vi "autonSample.vi"(0 "Auton Array":dbl[][](array[numeric]), 5 "MeasuredHeading":dbl, 9 "EncoderDistance":dbl) -> (4 "Left Drive":dbl(knob) scale=-1.0..1.0, 6 "Right Drive":dbl(knob) scale=-1.0..1.0, 8 "Ramp ACT motor":dbl, 10 "Turret Rotation":dbl, 13 "Conveyor":dbl, 14 "Harvester":dbl, 15 "Shooter motor output":dbl)   [LabVIEW 2011]
uses:
  Robot Global Data.vi
  <vilib>/addons/control/pid/pid.llb/PID (DBL).vi
  <vilib>/addons/control/pid/NI_PID_pid.lvlib
panel:
  out "Numeric":i16
  out "Tzero":i64
  out "AccumDist":dbl
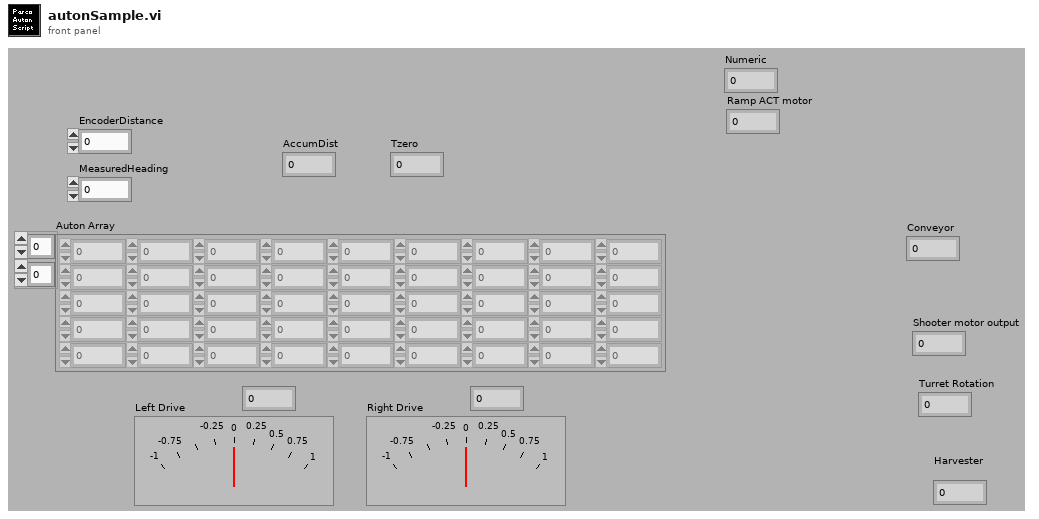
[diagram p1: front panel]
types:
  T1 = cluster{"proportional gain (Kc)":dbl, "integral time (Ti, min)":dbl, "derivative time (Td, min)":dbl}
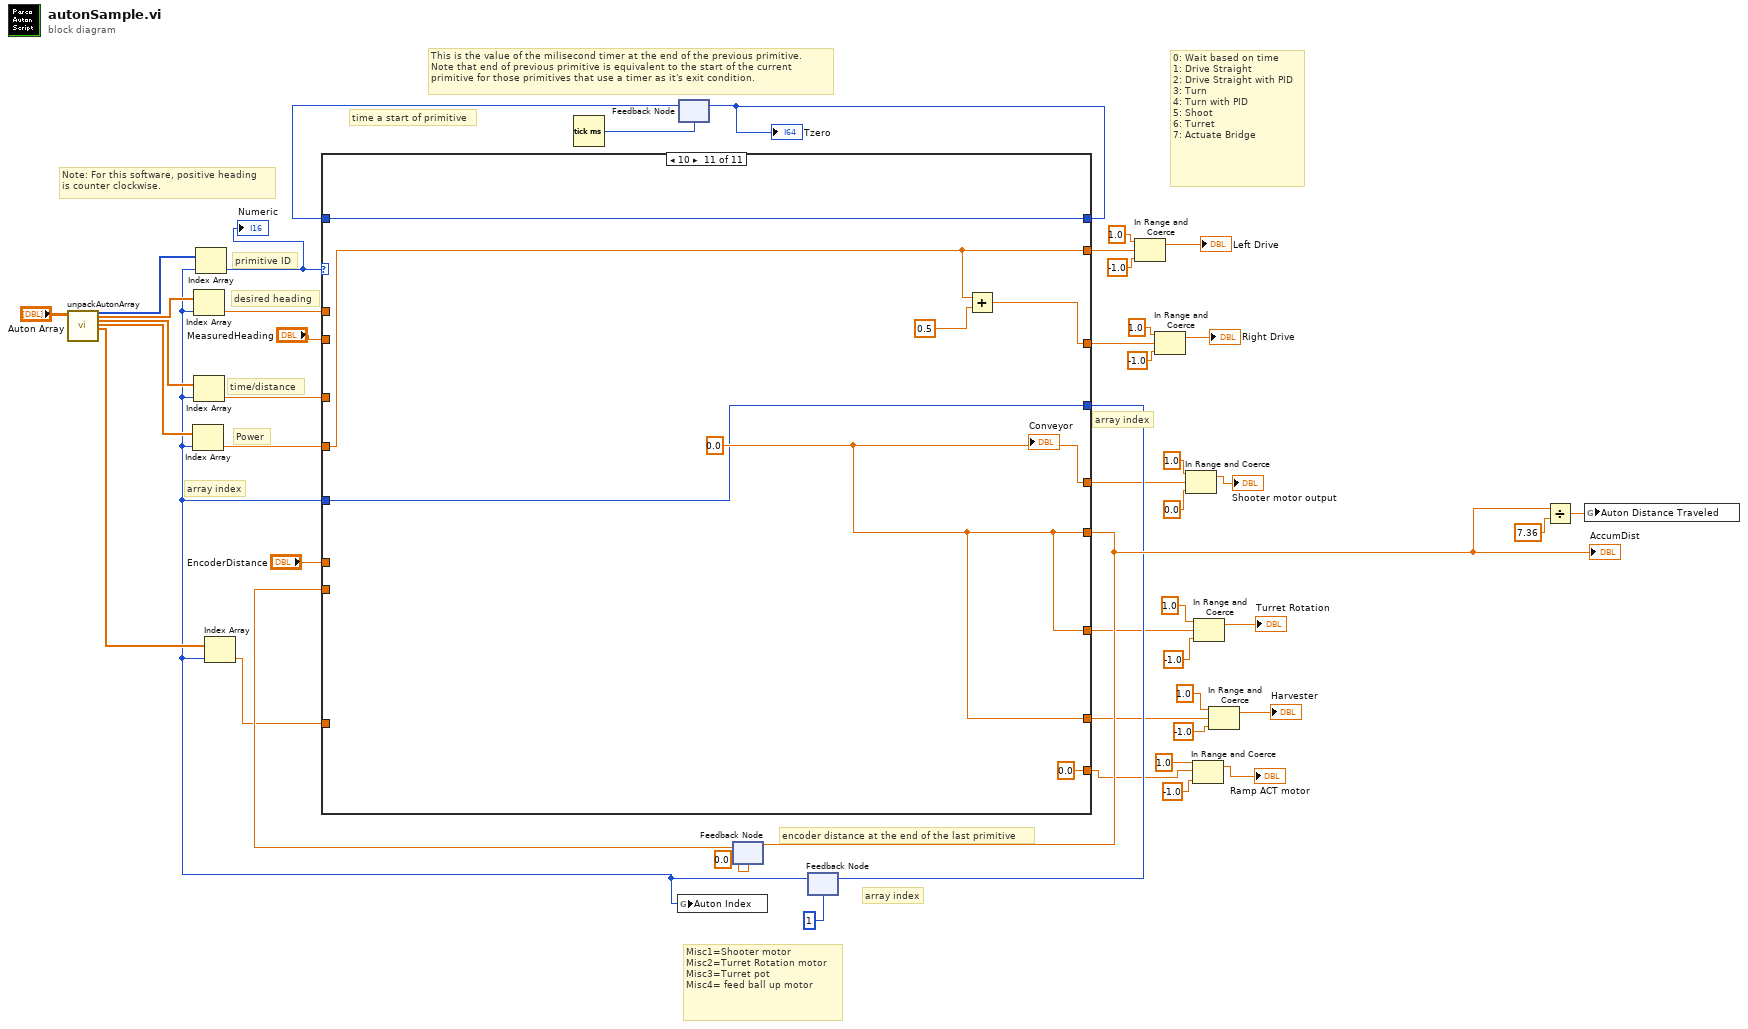
[diagram p0: block diagram]
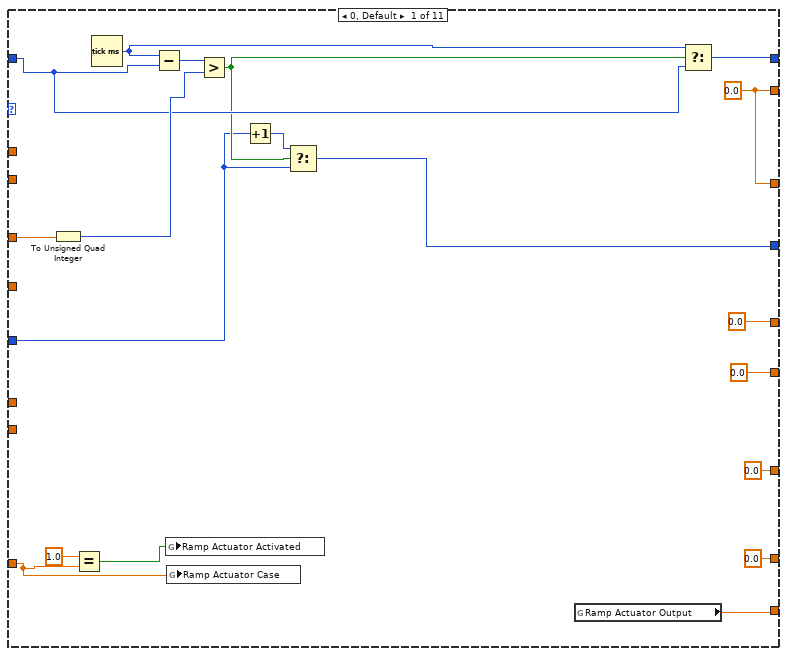
[diagram p2: hidden frame]
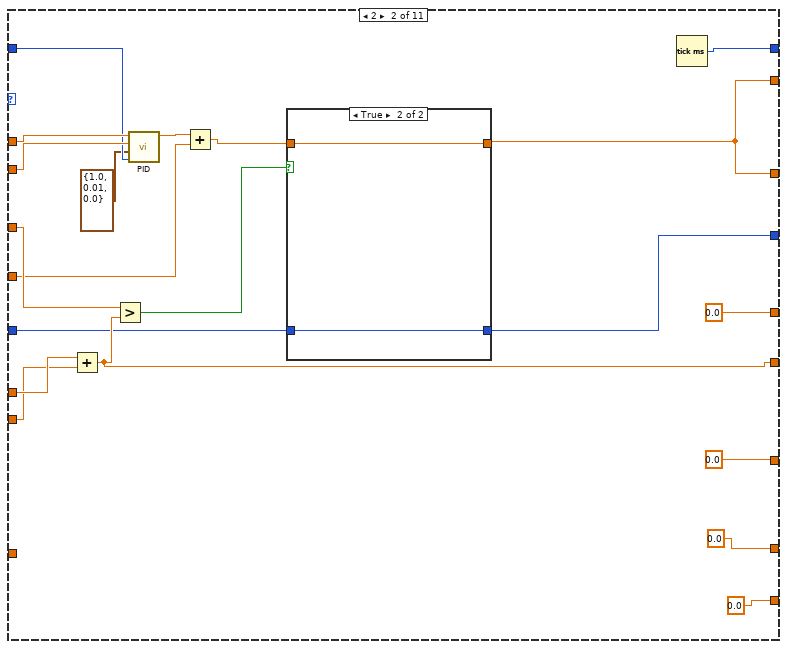
[diagram p3: hidden frame]
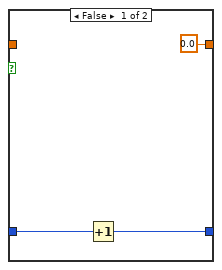
[diagram p4: hidden frame]
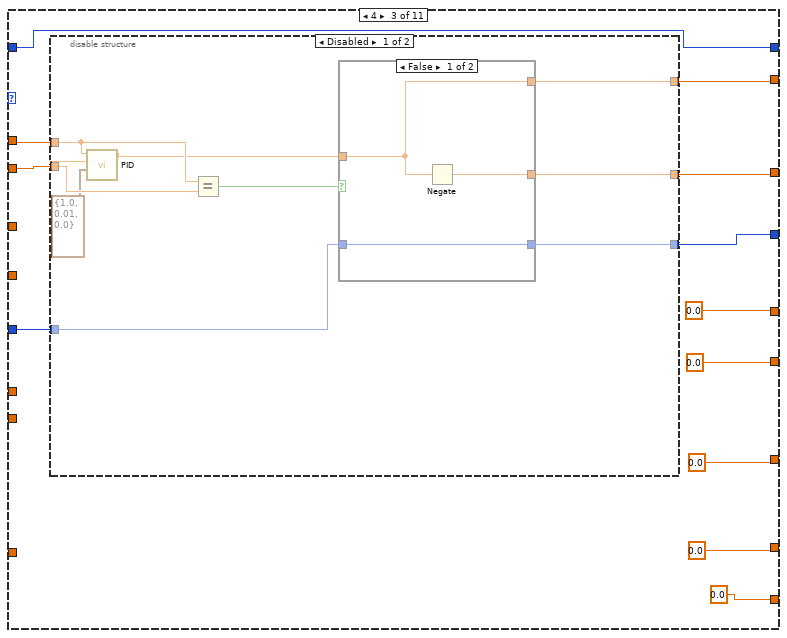
[diagram p5: hidden frame]
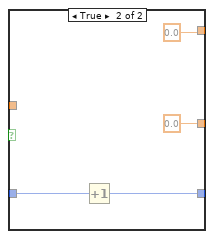
[diagram p6: hidden frame]
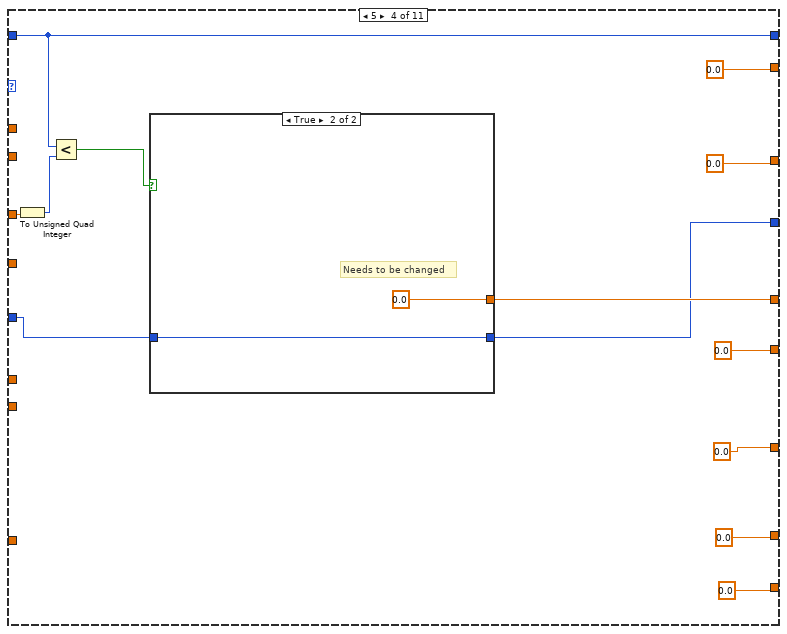
[diagram p8: hidden frame]
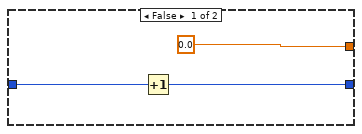
[diagram p9: hidden frame]
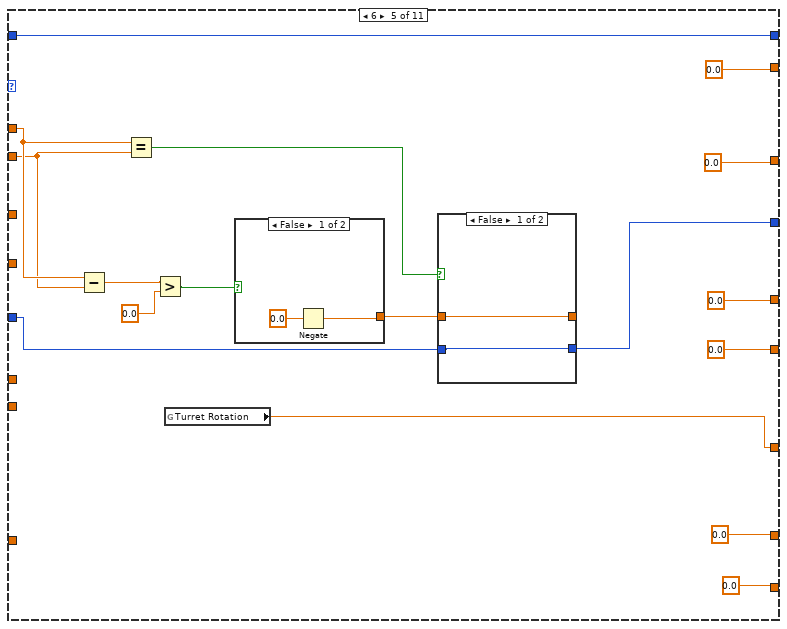
[diagram p10: hidden frame]
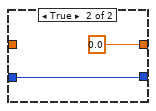
[diagram p11: hidden frame]
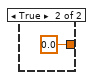
[diagram p12: hidden frame]
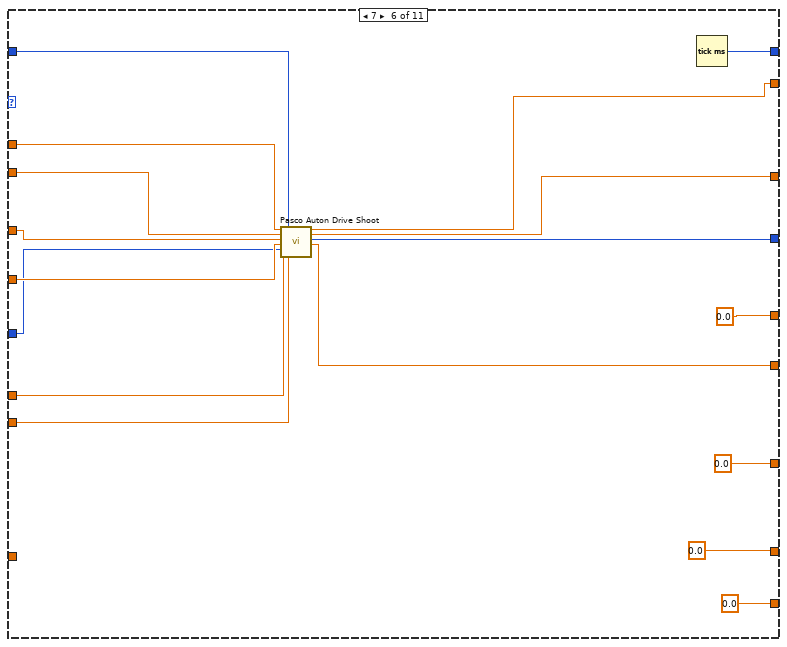
[diagram p13: hidden frame]
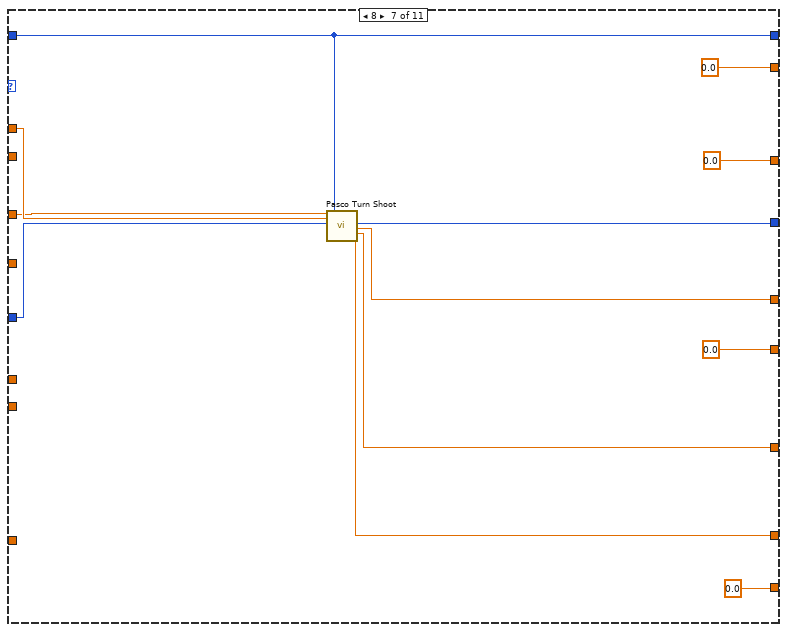
[diagram p14: hidden frame]
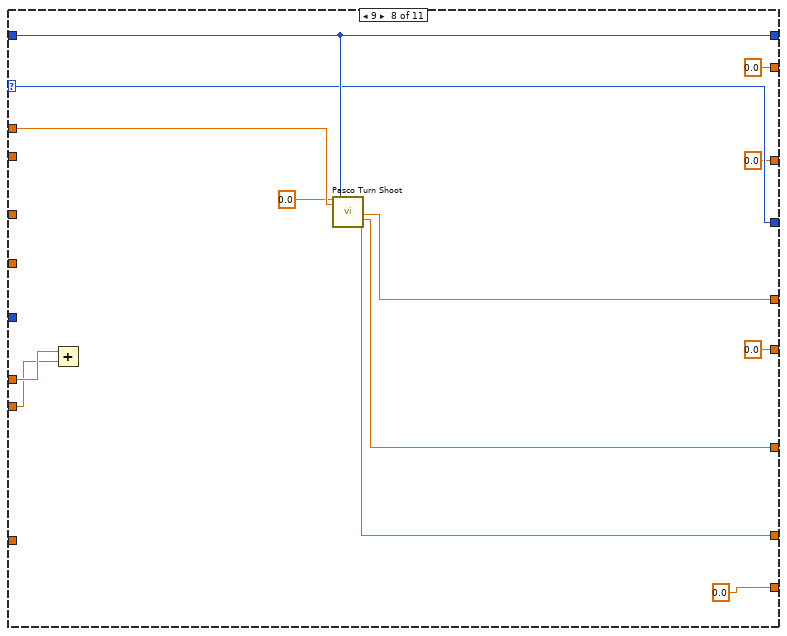
[diagram p15: hidden frame]
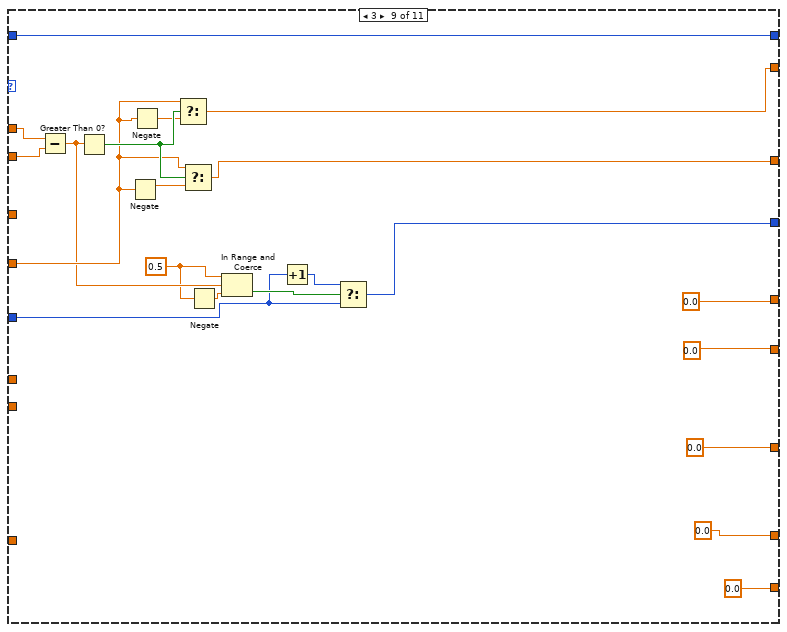
[diagram p16: hidden frame]
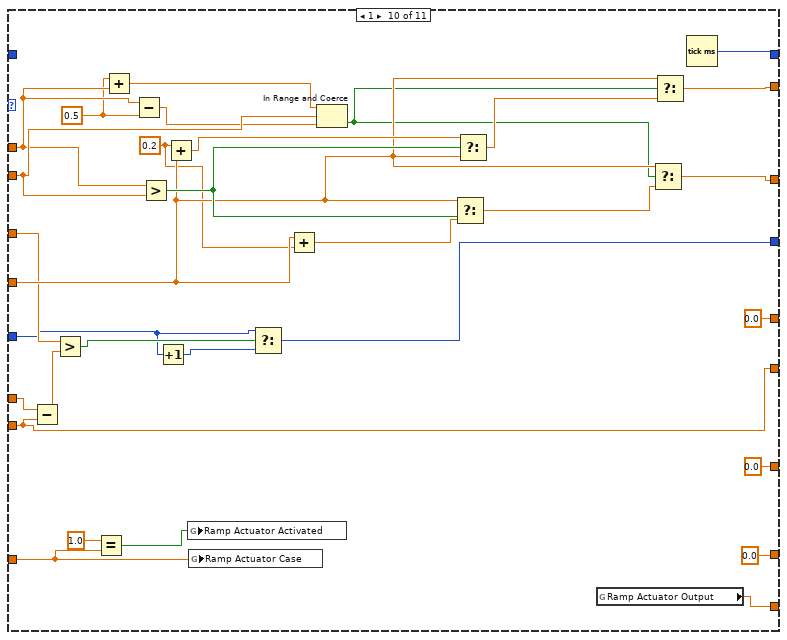
[diagram p17: hidden frame]
diagram:
  # "Misc1=Shooter motor\nMisc2=Turret Rotation motor\nMisc3=Turret pot\nMisc4= feed ball up motor"
  # "0: Wait based on time\n1: Drive Straight\n2: Drive Straight with PID\n3: Turn\n4: Turn with PID\n5: Shoot\n6: Turret\n7: Actuate Bridge"
  # "encoder distance at the end of the last primitive"
  # "Note: For this software, positive heading\nis counter clockwise."
  # "time a start of primitive"
  # "array index"
  # "array index"
  # "This is the value of the milisecond timer at the end of the previous primitive.\nNote that end of previous primitive is equivalent to the start of the current\nprimitive for those primitives that use a timer as it's exit condition."
  # "Power"
  # "array index"
  # "desired heading"
  # "primitive ID"
  # "time/distance"
  n1 = call "unpackAutonArray.vi"("all rows"="Auton Array") -> ("Primitive"=w47:i16[], "Left Drive"=w30:dbl[], "Right Drive"=w31:dbl[], "Ramp ACT"=w28:dbl[], "Conveyor"=w7:dbl[])  [unwired: 1 in, 21 out]
  n2 = Tick Count (ms)() -> (millisecond timer value=w42:u32)
  n3 = feedback #1(w42) -> (w46:u32)
  n4 = feedback #2(0.0 ("EncoderDistance")) -> (w27:dbl)
  n5 = feedback #3(1) -> (w6:i32)
  n6 = Index Array(array=w28, index=w6) -> (element=w44:dbl)
  n7 = Index Array(array=w30, index=w6) -> (element=w29:dbl)
  n8 = Index Array(array=w31, index=w6) -> (element=w45:dbl)
  n9 = Index Array(array=w47, index=w6) -> (element=w8:i16)
  "Numeric" <- w8
  n10 = Index Array(array=w7, index=w6) -> (element=w5:dbl)
  n11 = case shown="10" w8 {
    selector: w8 -> [_ _ _ _ _ _ _ w195 _ _ _]
    tunnel: [w55 w80 w98 w128 w151 w164 w188 w195 w207 w236 w262] -> w22
    tunnel: w6 -> [w56 w81 w97 w129 w152 w171 w191 _ w209 w234 w262]
    tunnel: [w67 w87 w104 w123 w150 w177 w189 w199 w205 w255 w261] -> w32
    tunnel: w46 -> [w63 w74 w104 w123 w150 w168 w189 w199 w205 _ w261]
    tunnel: w45 -> [w65 w83 _ w133 _ w173 w185 _ _ w238 _]
    tunnel: w29 -> [_ w75 w94 _ w155 w175 w190 w202 w221 w248 _]
    tunnel: [w54 w82 w99 0.0 0.0 w167 0.0 0.0 ("Numeric") w215 w239 w259] -> w40
    tunnel: [w54 w82 w100 0.0 0.0 w166 0.0 0.0 ("Right Drive") w214 w240 w258] -> w33
    tunnel: w44 -> [_ w71 _ _ _ w172 _ _ w217 w243 w259]
    tunnel: "EncoderDistance" -> [_ w86 _ _ _ w169 _ w204 _ w233 _]
    tunnel: "MeasuredHeading" -> [_ w76 w95 _ w141 w174 _ _ w220 w249 _]
    tunnel: [0.0 ("Encoder total") w84 0.0 0.0 0.0 w165 0.0 0.0 ("Encoder total") 0.0 w231 w263] -> w24
    tunnel: w27 -> [_ w85 _ _ _ w170 _ w203 _ w231 _]
    tunnel: [0.0 ("Misc1  OUT") 0.0 0.0 w130 0.0 0.0 ("Misc1  OUT") w187 w201 0.0 0.0 ("Misc1  OUT") w263] -> w18
    tunnel: [0.0 ("Misc2 OUT") 0.0 0.0 0.0 w140 0.0 ("Misc1  OUT") w186 w200 0.0 0.0 ("Misc2 OUT") w263] -> w14
    tunnel: [0.0 ("Misc4 OUT") 0.0 0.0 0.0 0.0 0.0 w181 w197 0.0 0.0 w263] -> w10
    tunnel: w5 -> [w50 _ _ _ _ _ _ _ _ w229 _]
    tunnel: [w49 0.0 ("Ramp Actuator Output") 0.0 ("Ramp Actuator Output") 0.0 ("Ramp Actuator Output") 0.0 ("Ramp Actuator Output") 0.0 ("Ramp Actuator Output") 0.0 ("Ramp Actuator Output") 0.0 ("Ramp Actuator Output") 0.0 ("Ramp Actuator Output") w226 0.0 ("Ramp Actuator Output")] -> w4
    frame 0, Default {
      w54 = 0.0 ("Numeric")
      n12 = To Unsigned Quad Integer(1:w65) -> (0:w64:u64)
      n13 = Equal?(x=1.0, y=w50) -> (x = y?=w51:bool)
      n14 = Tick Count (ms)() -> (millisecond timer value=w62:u32)
      n15 = Subtract(x=w62, y=w63) -> (x-y=w66:u32)
      n16 = global write "Robot Global Data.vi" "Ramp Actuator Activated"(w51) -> ()
      n17 = global write "Robot Global Data.vi" "Ramp Actuator Case"(w50) -> ()
      n18 = Greater?(x=w66, y=w64) -> (0:w58:bool)
      n19 = Increment(x=w56) -> (x+1=w57:i32)
      n20 = Select(t=w57, s=w58, f=w56) -> (s? t:f=w55:i32)
      n21 = global read "Robot Global Data.vi" "Ramp Actuator Output"() -> (w49:dbl)
      n22 = Select(t=w62, s=w58, f=w63) -> (s? t:f=w67:u32)
    }
    frame 2 {
      n23 = Add(x=w86, y=w85) -> (x+y=w84:dbl)
      n24 = Greater?(x=w83, y=w84) -> (0:w73:bool)
      n25 = call-poly <vilib>:"PID.vi"("dt (s)"=w74, "PID gains"=T1 {"proportional gain (Kc)"=1.0, "integral time (Ti, min)"=0.01, "derivative time (Td, min)"=0.0}, "process variable"=w76, "setpoint"=w75) -> ("output"=w70:dbl)  [unwired: 6 in, 1 out]
      n26 = Add(x=w70, y=w71) -> (x+y=w69:dbl)
      n27 = case shown="True" w73 {
        tunnel: [0.0 w92] -> w82
        tunnel: w69 -> [_ w92]
        tunnel: w81 -> [w90 w91]
        tunnel: [w89 w91] -> w80
        frame False {
          n28 = Increment(x=w90) -> (x+1=w89:i32)
        }
        frame True {
        }
      }
      n29 = Tick Count (ms)() -> (millisecond timer value=w87:u32)
    }
    frame 4 {
      n30 = disable-structure shown="Disabled" {
        disable-tunnel: [w113 _] -> w100
        disable-tunnel: [w112 _] -> w99
        disable-tunnel: [w111 _] -> w98
        disable-tunnel: w97 -> [w110 _]
        disable-tunnel: w95 -> [w108 _]
        disable-tunnel: w94 -> [w107 _]
        frame Disabled {
          n31 = call-poly <vilib>:"PID.vi"("PID gains"=T1 {"proportional gain (Kc)"=1.0, "integral time (Ti, min)"=0.01, "derivative time (Td, min)"=0.0}, "process variable"=w108, "setpoint"=w107) -> ("output"=w106:dbl)  [unwired: 7 in, 1 out]
          n32 = Equal?(x=w107, y=w108) -> (x = y?=w109:bool)
          n33 = case shown="False" w109 {
            tunnel: w106 -> [w115 _]
            tunnel: [w116 0.0] -> w113
            tunnel: [w115 0.0] -> w112
            tunnel: [w114 w119] -> w111
            tunnel: w110 -> [w114 w120]
            frame False {
              n34 = Negate(x=w115) -> (-x=w116:dbl)
            }
            frame True {
              n35 = Increment(x=w120) -> (x+1=w119:i32)
            }
          }
        }
        frame Enabled {
        }
      }
    }
    frame 5 {
      n36 = To Unsigned Quad Integer(1:w133) -> (0:w131:u64)
      n37 = Less?(x=w123, y=w131) -> (x < y?=w132:bool)
      n38 = case shown="True" w132 {
        tunnel: [0.0 0.0] -> w130
        tunnel: w129 -> [w135 w138]
        tunnel: [w134 w138] -> w128
        frame False {
          n39 = Increment(x=w135) -> (x+1=w134:i32)
        }
        frame True {
          # "Needs to be changed"
        }
      }
    }
    frame 6 {
      n40 = Subtract(x=w155, y=w141) -> (x-y=w143:dbl)
      n41 = Equal?(x=w155, y=w141) -> (x = y?=w154:bool)
      n42 = Greater?(x=w143, y=0.0) -> (0:w144:bool)
      n43 = global read "Robot Global Data.vi" "Turret Rotation"() -> (w140:dbl)
      n44 = case shown="False" w144 {
        tunnel: [w161 0.0] -> w153
        frame False {
          n45 = Negate(x=0.0) -> (-x=w161:dbl)
        }
        frame True {
        }
      }
      n46 = case shown="False" w154 {
        tunnel: [w157 0.0] -> _
        tunnel: w153 -> [w157 _]
        tunnel: w152 -> [w156 w159]
        tunnel: [w156 w159] -> w151
        frame False {
        }
        frame True {
        }
      }
    }
    frame 7 {
      n47 = call "Pasco Auton Drive Shoot.vi"("Desired Heading"=w175, "Actual Heading"=w174, "time/distance"=w173, "Power"=w172, "Array"=w171, "Encoder total"=w169, "Time"=w168, "Encoder Return"=w170) -> ("Left Drive"=w167:dbl, "Right Drive"=w166:dbl, "Array Out"=w164:i32, "Encoder total"=w165:dbl)  [unwired: 8 in]
      n48 = Tick Count (ms)() -> (millisecond timer value=w177:u32)
    }
    frame 8 {
      n49 = call "Pasco Turn Shoot.vi"("time/distance"=w185, "desired heading"=w190, "array index"=w191, "primitive time"=w189) -> ("array index"=w188:i32, "Misc1  OUT"=w187:dbl, "Misc2 OUT"=w186:dbl, "Misc4 OUT"=w181:dbl)  [unwired: 12 in]
    }
    frame 9 {
      n50 = Add(x=w204, y=w203) -> ()  [unwired: 1 out]
      n51 = call "Pasco Turn Shoot.vi"("time/distance"=0.0, "desired heading"=w202, "primitive time"=w199) -> ("Misc1  OUT"=w201:dbl, "Misc2 OUT"=w200:dbl, "Misc4 OUT"=w197:dbl)  [unwired: 13 in, 1 out]
    }
    frame 3 {
      w212 = 0.5 ("upper limit")
      n52 = Subtract(x=w221, y=w220) -> (x-y=w213:dbl)
      n53 = Greater Than 0?(x=w213) -> (x > 0?=w219:bool)
      n54 = Negate(x=w217) -> (-x=w218:dbl)
      n55 = Negate(x=w217) -> (-x=w216:dbl)
      n56 = Select(t=w217, s=w219, f=w216) -> (s? t:f=w215:dbl)
      n57 = Select(t=w217, s=w219, f=w218) -> (s? t:f=w214:dbl)
      n58 = Negate(x=w212) -> (-x=w211:dbl)
      n59 = In Range and Coerce(upper limit=w212, x=w213, lower limit=w211) -> (In Range?=w210:bool)  [unwired: 1 out]
      n60 = Increment(x=w209) -> (x+1=w208:i32)
      n61 = Select(t=w208, s=w210, f=w209) -> (s? t:f=w207:i32)
    }
    frame 1 {
      w247 = 0.5 ("x")
      w230 = 0.2 ("x")
      n62 = Subtract(x=w233, y=w231) -> (x-y=w232:dbl)
      n63 = Greater?(x=w238, y=w232) -> (0:w237:bool)
      n64 = Equal?(x=1.0, y=w229) -> (x = y?=w227:bool)
      n65 = Add(x=w247, y=w248) -> (x+y=w245:dbl)
      n66 = Subtract(x=w248, y=w247) -> (x-y=w246:dbl)
      n67 = Greater?(x=w248, y=w249) -> (0:w251:bool)
      n68 = Increment(x=w234) -> (x+1=w235:i32)
      n69 = Add(x=w230, y=w243) -> (x+y=w252:dbl)
      n70 = global write "Robot Global Data.vi" "Ramp Actuator Activated"(w227) -> ()
      n71 = global write "Robot Global Data.vi" "Ramp Actuator Case"(w229) -> ()
      n72 = Select(t=w234, s=w237, f=w235) -> (s? t:f=w236:i32)
      n73 = Add(x=w243, y=w230) -> (x+y=w250:dbl)
      n74 = In Range and Coerce(upper limit=w245, x=w249, lower limit=w246) -> (In Range?=w242:bool)  [unwired: 1 out]
      n75 = Select(t=w243, s=w251, f=w250) -> (s? t:f=w241:dbl)
      n76 = Select(t=w252, s=w251, f=w243) -> (s? t:f=w244:dbl)
      n77 = global read "Robot Global Data.vi" "Ramp Actuator Output"() -> (w226:dbl)
      n78 = Select(t=w243, s=w242, f=w241) -> (s? t:f=w240:dbl)
      n79 = Select(t=w243, s=w242, f=w244) -> (s? t:f=w239:dbl)
      n80 = Tick Count (ms)() -> (millisecond timer value=w255:u32)
    }
    frame 10 {
      w263 = 0.0
      n81 = Add(x=w259, y=0.5 ("x+y")) -> (x+y=w258:dbl)
    }
  }
  "AccumDist" <- w24
  "Tzero" <- w32
  n82 = global write "Robot Global Data.vi" "Auton Index"(w6) -> ()
  n83 = feedback-in #1(w32) -> ()
  n84 = feedback-in #2(w24) -> ()
  n85 = feedback-in #3(w22) -> ()
  n86 = In Range and Coerce(upper limit=1.0, x=w40, lower limit=-1.0) -> (coerced(x)=→"Left Drive":dbl)  [unwired: 1 out]
  n87 = In Range and Coerce(upper limit=1.0, x=w33, lower limit=-1.0) -> (coerced(x)=→"Right Drive":dbl)  [unwired: 1 out]
  n88 = In Range and Coerce(upper limit=1.0, x=w18, lower limit=0.0) -> (coerced(x)=→"Shooter motor output":dbl)  [unwired: 1 out]
  n89 = In Range and Coerce(upper limit=1.0, x=w4, lower limit=-1.0) -> (coerced(x)=→"Ramp ACT motor":dbl)  [unwired: 1 out]
  n90 = In Range and Coerce(upper limit=1.0, x=w14, lower limit=-1.0) -> (coerced(x)=→"Turret Rotation":dbl)  [unwired: 1 out]
  n91 = In Range and Coerce(upper limit=1.0, x=w10, lower limit=-1.0) -> (coerced(x)=→"Harvester":dbl)  [unwired: 1 out]
  n92 = Divide(x=w24, y=7.36) -> (x/y=w9:dbl)
  n93 = global write "Robot Global Data.vi" "Auton Distance Traveled"(w9) -> ()
